vi "Test STOMP Publish Subscribe.vi"() -> ()   [LabVIEW 2017]
uses:
  Typedefs/Type_ServerFrame.ctl
  Typedefs/Type_ServerFrameType.ctl
  Typedefs/Type_AckHeader.ctl
  STOMP.lvclass
  Typedefs/Type_FrameHeader.ctl
panel:
  in  "ack":T1
  in  "ACK?":bool
  out "error IO":errorcluster
  in  "Subscription Id":u64
  out "error out":errorcluster
  in  "Unsub":bool
  in  "Send":bool
  out "value":dbl[](array[numeric])
  out "Count":i32
  out "timed out?":bool
  out "receive error":errorcluster
  out "message":T2
  out "send error":errorcluster
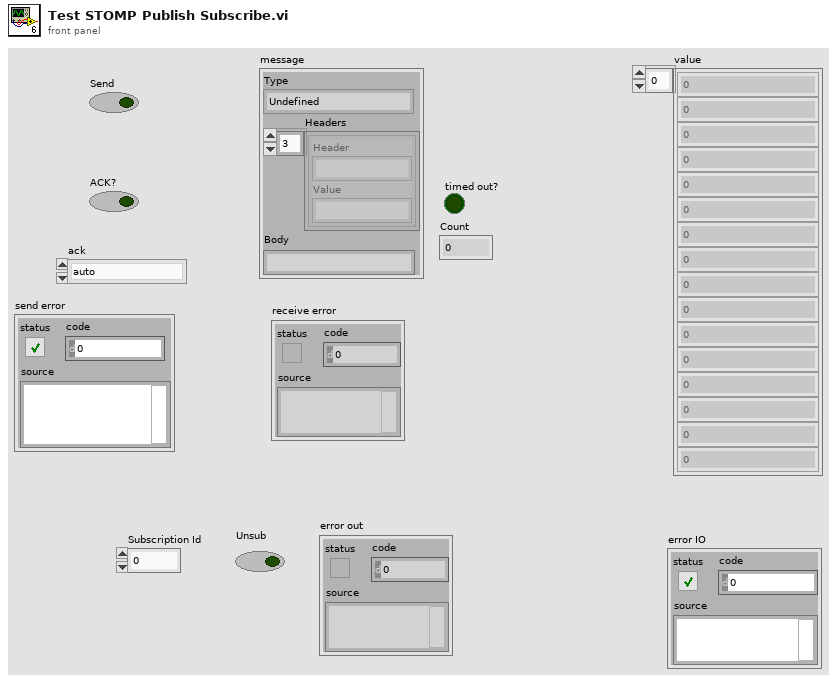
[diagram p1: front panel]
types:
  T1 = typedef "STOMP.lvclass/Type_AckHeader.ctl" = enum16{"auto", "client", "client-individual"}
  T2 = typedef "STOMP.lvclass/Type_ServerFrame.ctl" = cluster{"Type":T3, "Headers":cluster{"Header":string, "Value":string}[], "Body":string}
  T3 = typedef "STOMP.lvclass/Type_ServerFrameType.ctl" = enum16{"Undefined", "MESSAGE", "CONNECTED", "RECEIPT", "ERROR"}
  T4 = typedef "STOMP.lvclass/Type_FrameHeader.ctl" = cluster{"Header":string, "Value":string}
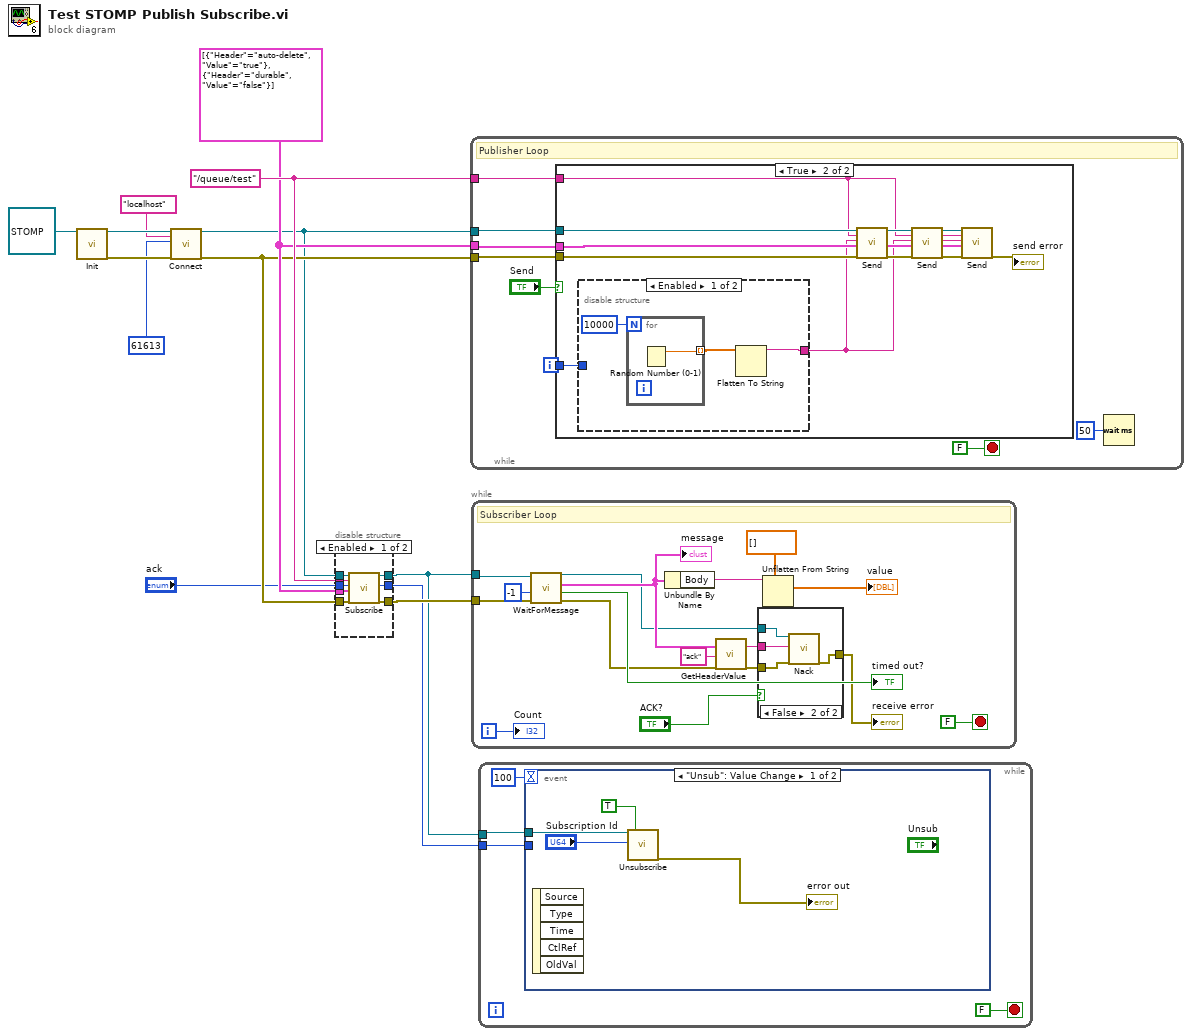
[diagram p0: block diagram]
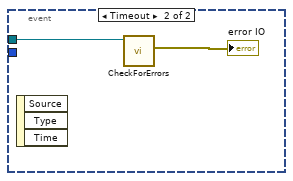
[diagram p2: hidden frame]
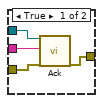
[diagram p4: hidden frame]
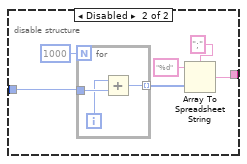
[diagram p6: hidden frame]
diagram:
  w7 = T4[] [{"Header"="auto-delete", "Value"="true"}, {"Header"="durable", "Value"="false"}] ("headers")
  w8 = "/queue/test" ("Destination")
  n1 = call "Init.vi"("STOMP in"=refnum<class "STOMP.lvclass"> refnum) -> ("STOMP out"=w12:refnum<class "STOMP.lvclass">, "error out"=w13:errorcluster)  [unwired: 17 in]
  n2 = call "Connect.vi"("STOMP in"=w12, "address"="localhost", "port"=u16 61613, "error in"=w13) -> ("STOMP out"=w5:refnum<class "STOMP.lvclass">, "error out"=w6:errorcluster)  [unwired: 14 in]
  n3 = disable-structure shown="Enabled" {
    disable-tunnel: [w21 w23] -> w2
    disable-tunnel: [w20 w22] -> w4
    disable-tunnel: w8 -> [w19 _]
    disable-tunnel: w7 -> [w18 _]
    disable-tunnel: w6 -> [w17 w22]
    disable-tunnel: w5 -> [w16 w23]
    disable-tunnel: [w15 _] -> w3
    disable-tunnel: "ack" -> [w14 _]
    frame Enabled {
      n4 = call-dynamic "Subscribe.vi"("STOMP in"=w16, "Destination"=w19, "ack"=w14, "headers"=w18, "error in (no error)"=w17) -> ("STOMP out"=w21:refnum<class "STOMP.lvclass">, "Subscription ID"=w15:u64, "error out"=w20:errorcluster)  [unwired: 12 in]
    }
    frame Disabled {
    }
  }
  n5 = while {
    tunnel: w5 -> [w31]
    tunnel: w8 -> [w25]
    tunnel: w6 -> [w30]
    tunnel: w7 -> [w26]
    i -> [w27]
    stop <- FALSE stop-if-true
    # "Publisher Loop"
    n6 = case shown="True" "Send" {
      tunnel: w31 -> [_ w42]
      tunnel: w30 -> [_ w41]
      tunnel: w27 -> [_ w40]
      tunnel: w26 -> [_ w37]
      tunnel: w25 -> [_ w35]
      frame False {
      }
      frame True {
        n7 = disable-structure shown="Enabled" {
          disable-tunnel: [w43 w47] -> w36
          disable-tunnel: w40 -> [_ w48]
          frame Enabled {
            n8 = for {
              N: 10000 -> [_]
              tunnel: [w46] -> w44 mode=indexing
              n9 = Random Number (0-1)() -> (number: 0 to 1=w46:dbl)
            }
            n10 = Flatten To String(anything=w44) -> (data string=w43:string)  [unwired: 3 in, 2 out]
          }
          frame Disabled {
            n11 = for {
              N: 1000 -> [_]
              tunnel: w48 -> [w55]
              tunnel: [w53] -> w51 mode=indexing
              i -> [w54]
              n12 = Add(x=w54, y=w55) -> (x+y=w53:i32)
            }
            n13 = Array To Spreadsheet String(delimiter (Tab)=";", array=w51, 3:"%d" ("format string")) -> (spreadsheet string=w47:string)
          }
        }
        n14 = call-dynamic "Send.vi"("STOMP in"=w42, "Destination"=w35, "Body"=w36, "headers"=w37, "error in (no error)"=w41) -> ("STOMP out"=w39:refnum<class "STOMP.lvclass">, "error out"=w38:errorcluster)  [unwired: 13 in]
        n15 = call-dynamic "Send.vi"("STOMP in"=w39, "Destination"=w35, "Body"=w36, "headers"=w37, "error in (no error)"=w38) -> ("STOMP out"=w34:refnum<class "STOMP.lvclass">, "error out"=w33:errorcluster)  [unwired: 13 in]
        n16 = call-dynamic "Send.vi"("STOMP in"=w34, "Destination"=w35, "Body"=w36, "headers"=w37, "error in (no error)"=w33) -> ("error out"=→"send error":errorcluster)  [unwired: 13 in, 1 out]
      }
    }
    n17 = Wait (ms)(milliseconds to wait=u32 50) -> ()  [unwired: 1 out]
  }
  n18 = while {
    tunnel: w2 -> [w72]
    tunnel: w4 -> [w71]
    i -> [w67]
    stop <- FALSE stop-if-true
    # "Subscriber Loop"
    n19 = call-dynamic "WaitForMessage.vi"("error in (no error)"=w71, "timeout in ms (10000)"=-1, "STOMP in"=w72) -> ("error out"=w60:errorcluster, "timed out?"=→"timed out?":bool, "message"=w63:T2, "STOMP out"=w59:refnum<class "STOMP.lvclass">)  [unwired: 5 in]
    "message" <- w63
    n20 = Unbundle By Name(w63) -> ("Body"=w66:string)
    n21 = call "GetHeaderValue.vi"("Server Frame"=w63, "Header Name"="ack", "error in"=w60) -> ("Value"=w58:string, "error out"=w61:errorcluster)  [unwired: 14 in, 1 out]
    n22 = case shown="False" "ACK?" {
      tunnel: w61 -> [w76 w80]
      tunnel: w59 -> [w75 w79]
      tunnel: w58 -> [w74 w78]
      tunnel: [w73 w77] -> w57
      frame True {
        n23 = call "Ack.vi"("STOMP in"=w75, "ack id"=w74, "error in (no error)"=w76) -> ("error out"=w73:errorcluster)  [unwired: 15 in, 1 out]
      }
      frame False {
        n24 = call-dynamic "Nack.vi"("STOMP in"=w79, "ack id"=w78, "error in (no error)"=w80) -> ("error out"=w77:errorcluster)  [unwired: 15 in, 1 out]
      }
    }
    "receive error" <- w57
    n25 = Unflatten From String(type=dbl[] [], binary string=w66) -> (value=→"value":dbl[])  [unwired: 3 in, 2 out]
    "Count" <- w67
  }
  n26 = while {
    tunnel: w3 -> [w82]
    tunnel: w2 -> [w83]
    stop <- FALSE stop-if-true
    n27 = event shown="[0] \"Unsub\": Value Change" {
      selector: _ -> [_ _]
      dyn-events: _ -> [_ _]
      timeout: 100 -> [_ _]
      tunnel: w83 -> [w88 w90]
      tunnel: w82 -> [_ _]
      event "Unsub": Value Change {
        n28 = event-data() -> ()  [unwired: 1 in, 5 out]
        n29 = call-dynamic "Unsubscribe.vi"("STOMP in"=w88, "Subscription Id"="Subscription Id", "Receipt?"=TRUE) -> ("error out"=→"error out":errorcluster)  [unwired: 15 in, 1 out]
      }
      event Timeout {
        n30 = event-data() -> ()  [unwired: 1 in, 3 out]
        n31 = call-dynamic "CheckForErrors.vi"("STOMP in"=w90) -> ("stomp error msg"=→"error IO":errorcluster)  [unwired: 8 in, 2 out]
      }
    }
  }
